vi "Get TD Header Subset.vi"(8 "错误输入（无错误）":errorcluster, 11 "Variant":variant) -> (0 "错误输出":errorcluster, 2 "Data String":string, 3 "Type Descriptor Head Subset":u16[](array[numeric]))   [LabVIEW 2012, in "TD Tools.lvlib"]
uses:
  TD Tools.lvlib
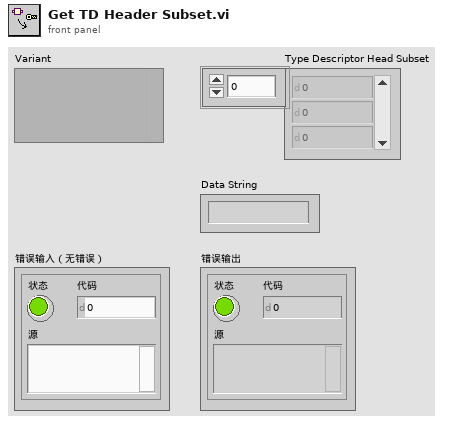
[diagram p1: front panel]
types:
  T1 = typedef "TD Tools.lvlib/Type Descriptor.ctl" = u16[]
  T2 = typedef "TD Tools.lvlib/Type Descriptor Header.ctl" = cluster{"length":u16, "private":u8, "type":T3, "# elements":u16}
  T3 = typedef "TD Tools.lvlib/Type Descriptor Enumeration.ctl" = enum16{"<Null>", "I8", "I16", "I32", "I64", "U8", "U16", "U32", "U64", "SGL", "DBL", "EXT", "CSG", "CDB", "CXT", "0x0F", "0x10", "0x11", "0x12", "0x13", "0x14", "Enum U8", "Enum U16", "Enum U32", "Enum U64", "SGL PQ", "DBL PQ", "EXT PQ", "CSG PQ", "CDB PQ", "CXT PQ", "0x1F", "0x20", "Boolean", "0x22", "0x23", "0x24", "0x25", "0x26", "0x27", "0x28", "0x29", "0x2A", "0x2B", "0x2C", "0x2D", "0x2E", "0x2F", "String", "0x31", "Path", "Pict", "0x34", "0x35", "0x36", "DAQ", "0x38", "0x39", "0x3A", "0x3B", "0x3C", "0x3D", "0x3E", "0x3F", "Array", "0x41", "0x42", "0x43", "0x44", "0x45", "0x46", "0x47", "0x48", "0x49", "0x4A", "0x4B", "0x4C", "0x4D", "0x4E", "0x4F", "Cluster", "0x51", "0x52", "Variant", "Waveform", "0x55", "0x56", "0x57", "0x58", "0x59", "0x5A", "0x5B", "0x5C", "0x5D", "0x5E", "0x5F", "0x60", "0x61", "0x62", "0x63", "0x64", "0x65", "0x66", "0x67", "0x68", "0x69", "0x6A", "0x6B", "0x6C", "0x6D", "0x6E", "0x6F", "Refnum"}
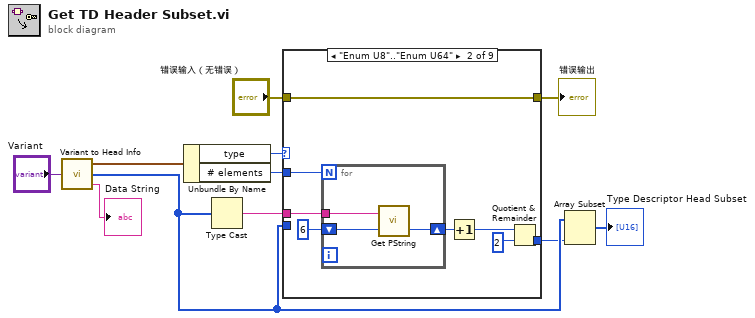
[diagram p0: block diagram]
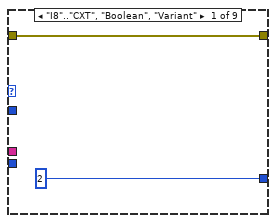
[diagram p2: hidden frame]
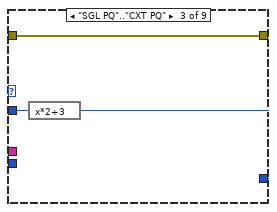
[diagram p3: hidden frame]
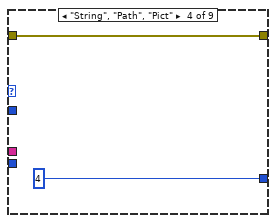
[diagram p4: hidden frame]
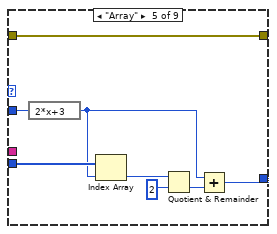
[diagram p5: hidden frame]
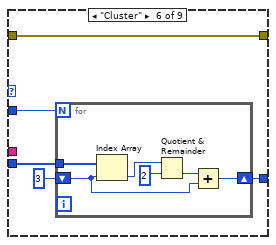
[diagram p6: hidden frame]
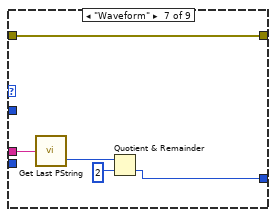
[diagram p7: hidden frame]
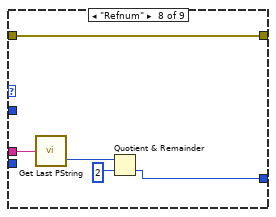
[diagram p8: hidden frame]
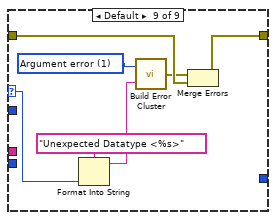
[diagram p9: hidden frame]
diagram:
  n1 = call "Variant to Head Info.vi"("Variant"="Variant") -> ("Data String"=→"Data String":string, "Type Descriptor"=w9:T1, "Type Descriptor Header"=w1:T2)  [unwired: 2 in]
  n2 = Unbundle By Name(w1) -> ("type"=w2:T3, "# elements"=w4:u16)
  n3 = Type Cast(x=w9) -> (*(type *) &x=w3:string)  [unwired: 1 in]
  n4 = case shown="\"Enum U8\"..\"Enum U64\"" w2 {
    selector: w2 -> [_ _ _ _ _ _ _ _ w63]
    tunnel: [w12 w15 w25 w28 w30 w38 w49 w54 w59] -> w8
    tunnel: w3 -> [_ w14 _ _ _ _ w53 w58 _]
    tunnel: w4 -> [_ w19 w27 _ w37 w42 _ _ _]
    tunnel: w9 -> [_ _ _ _ w36 w41 _ _ _]
    tunnel: [2 ("offset (0)") w16 w26 4 ("offset (0)") w31 w39 w50 w55 _] -> w5
    tunnel: "错误输入（无错误）" -> [w12 w15 w25 w28 w30 w38 w49 w54 w61]
    frame "I8".."CXT", "Boolean", "Variant" {
    }
    frame "Enum U8".."Enum U64" {
      n5 = for {
        N: w19 -> [_]
        tunnel: w14 -> [w22]
        shift-right: [w23] -> w20
        shift-left: 6 -> [w24]
        n6 = call "Get PString.vi"("offset(0)"=w24, "String"=w22) -> ("offset  Past PString"=w23:i32)  [unwired: 1 out]
      }
      n7 = Increment(x=w20) -> (x+1=w17:i32)
      n8 = Quotient & Remainder(x=w17, y=2) -> (floor(x/y)=w16:i32)  [unwired: 1 out]
    }
    frame "SGL PQ".."CXT PQ" {
      n9 = expression code="x*2+3"(w27) -> (w26:u16)
    }
    frame "String", "Path", "Pict" {
    }
    frame "Array" {
      n10 = expression code="2*x+3"(w37) -> (w32:u16)
      n11 = Index Array(array=w36, index=w32) -> (element=w34:u16)
      n12 = Quotient & Remainder(x=w34, y=u16 2) -> (floor(x/y)=w33:u16)  [unwired: 1 out]
      n13 = Add(x=w32, y=w33) -> (x+y=w31:u16)
    }
    frame "Cluster" {
      n14 = for {
        N: w42 -> [_]
        shift-right: [w47] -> w39
        shift-left: i16 3 -> [w46]
        tunnel: w41 -> [w48]
        n15 = Index Array(array=w48, index=w46) -> (element=w44:u16)
        n16 = Quotient & Remainder(x=w44, y=i16 2) -> (floor(x/y)=w45:u16)  [unwired: 1 out]
        n17 = Add(x=w45, y=w46) -> (x+y=w47:u16)
      }
    }
    frame "Waveform" {
      n18 = call "Get Last PString.vi"("String"=w53) -> ("PString Offset"=w51:i32)  [unwired: 1 out]
      n19 = Quotient & Remainder(x=w51, y=2) -> (floor(x/y)=w50:i32)  [unwired: 1 out]
    }
    frame "Refnum" {
      n20 = call "Get Last PString.vi"("String"=w58) -> ("PString Offset"=w56:i32)  [unwired: 1 out]
      n21 = Quotient & Remainder(x=w56, y=2) -> (floor(x/y)=w55:i32)  [unwired: 1 out]
    }
    frame Default {
      w65 = 1 items=["No error", "Argument error", "Memory is full", "Out of zone", "End of file", "File already open", "Generic file I/O error", "File not found", "File permission error", "Disk is full", "Duplicate path", "Too many files open", "System feature not enabled", "Resource file not found", "Cannot add resource", "Resource not found", "Image not found", "Image memory error", "Pen does not exist", "Config type invalid", "Config token not found", "Config parse error", "Config memory error", "Bad external code format", "Bad external code offset", "External code not present", "Null window", "Destroy window error", "Null menu", "Print aborted", "Bad print record", "Print driver error", "Windows error during printing", "Memory error during printing", "Print dialog error", "Generic print error", "Invalid device refnum", "Device not found", "Device parameter error", "Device unit error", "Cannot open device", "Device call aborted", "Generic error", "Cancelled by user", "Object ID too low", "Object ID too high", "Object not in heap", "Unknown heap", "Unknown object (invalid DefProc)", "Unknown object (DefProc not in table)", "Message out of range", "Invalid (null) method", "Unknown message", "Manager call not supported", "Bad address", "Network operation in progress", "Network operation timed out", "Connection is busy", "Network attribute not supported", "Network error", "Address in use", "System out of memory", "Connection aborted", "Connection refused", "Not connected", "Already connected", "Connection closed", "Initialization error (interapplication manager)", "Bad occurrence", "Wait on unbound occurrence handler", "Occurrence queue overflow", "Datalog type conflict", "Unused", "Unrecognized type (interapplication manager)", "Memory corrupt", "Failed to make temporary DLL", "Old CIN version", "Drag socket not found", "Failed to load drop-object", "Failed to register OLE object", "Failed to release OLE object", "Format specifier type mismatch", "Unknown format specifier", "Too few format specifiers", "Too many format specifiers", "Scan failed", "Newer CIN version", "Error converting to variant", "Runtime menu error", "Password tampered", "Variant attribute not found", "Incompatible variant data type", "Event data is not available", "Event Store is not present", "Occurrence is not found", "Event Queue is not created", "Event info is not available", "Refnum passed is NULL", "Error retrieving Class GUID", "Error retrieving CoClass GUID", "Error retrieving TypeLib GUID.", "Bad built application magic bytes.", "Specific driver is different from the specific driver associated with the Logical Name.", "There is no session opened to the class driver.", "Max Error", "MAX - Error with config objects", "MAX - Error loading configuration", "MAX - Group not supported"]
      n22 = Format Into String(format string="Unexpected Datatype <%s>" ("Format String"), w63) -> (resulting string=w62:string)  [unwired: 2 in, 1 out]
      n23 = call "Build Error Cluster.vi"("String to Prepend to source (\"\")"=w62, "code"=w65) -> ("error out"=w60:errorcluster)
      n24 = Merge Errors(w60, w61) -> (w59:errorcluster)
    }
  }
  "错误输出" <- w8
  n25 = Array Subset(array=w9, length=w5) -> (→"Type Descriptor Head Subset":T1)  [unwired: 1 in]
